vi "Set Diverter.vi"(8 "error in (no error)":errorcluster, 9 "Diverter Port":T1, 10 "Diverter Location":T2, 11 "SpectraPro in":refnum<class "SpectraPro.lvclass">) -> (0 "error out":errorcluster, 1 "Diverter Port out":T1, 3 "SpectraPro out":refnum<class "SpectraPro.lvclass">)   [LabVIEW 2019, in "SpectraPro.lvclass"]
uses:
  SpectraPro.lvclass
  SpectraPro-LabVIEW-Driver/Libraries/Types/Diverter Location.ctl
  SpectraPro-LabVIEW-Driver/Libraries/Types/Diverter Port.ctl
  SpectraPro.lvclass/SpectraPro.ctl
  SpectraPro-LabVIEW-Driver/SpectraPro.lvlib
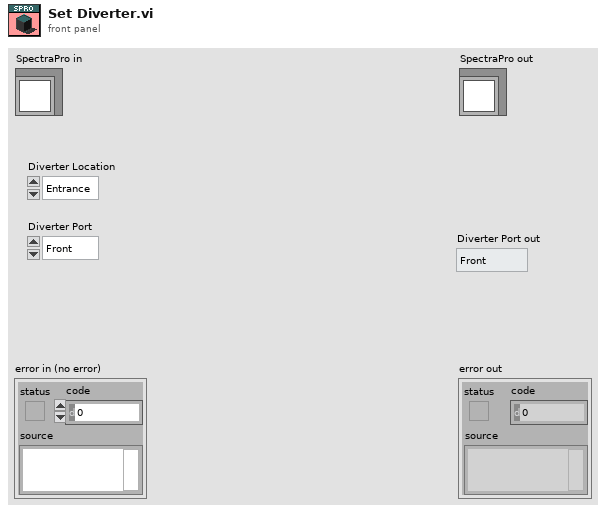
[diagram p1: front panel]
types:
  T1 = typedef "SpectraPro.lvlib/Diverter Port.ctl" = enum16{"Front", "Side"}
  T2 = typedef "Diverter Location.ctl" = enum16{"Entrance", "Exit"}
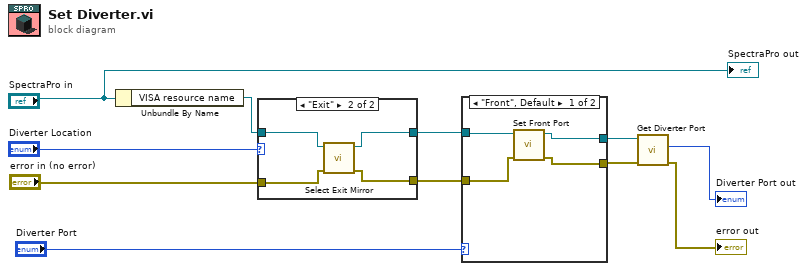
[diagram p0: block diagram]
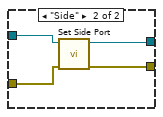
[diagram p2: hidden frame]
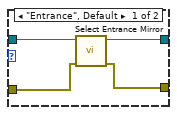
[diagram p3: hidden frame]
diagram:
  n1 = Unbundle By Name("SpectraPro in") -> ("VISA resource name"=w10:refnum<visa-resource-name>)
  n2 = case shown="\"Exit\"" "Diverter Location" {
    tunnel: w10 -> [w15 w19]
    tunnel: "error in (no error)" -> [w14 w17]
    tunnel: [w13 w16] -> w6
    tunnel: [w12 w18] -> w7
    frame "Entrance", Default {
      n3 = call "Select Entrance Mirror.vi"("error in (no error)"=w14, "VISA resource name"=w15) -> ("error out"=w13:errorcluster, "VISA resource name out"=w12:refnum<visa-resource-name>)  [unwired: 7 in, 1 out]
    }
    frame "Exit" {
      n4 = call "Select Exit Mirror.vi"("error in (no error)"=w17, "VISA resource name"=w19) -> ("error out"=w16:errorcluster, "VISA resource name out"=w18:refnum<visa-resource-name>)  [unwired: 7 in, 1 out]
    }
  }
  n5 = case shown="\"Front\", Default" "Diverter Port" {
    tunnel: w7 -> [w23 w27]
    tunnel: w6 -> [w21 w26]
    tunnel: [w22 w25] -> w5
    tunnel: [w20 w24] -> w2
    frame "Front", Default {
      n6 = call "Set Front Port.vi"("error in (no error)"=w21, "VISA resource name"=w23) -> ("error out"=w20:errorcluster, "VISA resource name out"=w22:refnum<visa-resource-name>)  [unwired: 7 in, 1 out]
    }
    frame "Side" {
      n7 = call "Set Side Port.vi"("error in (no error)"=w26, "VISA resource name"=w27) -> ("error out"=w24:errorcluster, "VISA resource name out"=w25:refnum<visa-resource-name>)  [unwired: 7 in, 1 out]
    }
  }
  n8 = call "Get Diverter Port.vi"("error in (no error)"=w2, "VISA resource name"=w5) -> ("error out"=→"error out":errorcluster, "Diverter Port"=→"Diverter Port out":T1)  [unwired: 6 in, 2 out]
  "SpectraPro out" <- "SpectraPro in"
